vi "getState.vi"(8 "error in (no error)":errorcluster, 11 "ReadingState in":refnum<class "ReadingState.lvclass">) -> (0 "error out":errorcluster, 2 "State":T1, 3 "ReadingState out":refnum<class "ReadingState.lvclass">)   [LabVIEW 2016, in "ReadingState.lvclass"]
uses:
  ReadingState.lvclass
  internalState.ctl
  Electrometer.lvclass
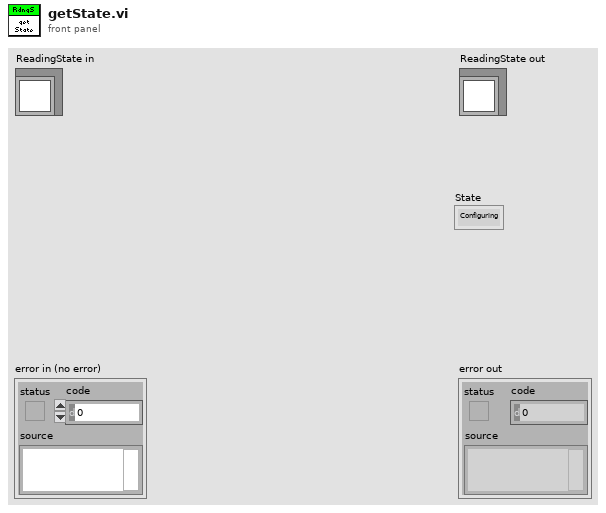
[diagram p1: front panel]
types:
  T1 = typedef "Electrometer.lvclass/internalState.ctl" = enum16{"Configuring", "Ready", "Reading"}
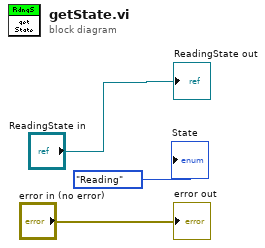
[diagram p0: block diagram]
diagram:
  "error out" <- "error in (no error)"
  "ReadingState out" <- "ReadingState in"
  "State" <- internalState."Reading" ("State")
